vi "Init Plot.vi"(8 "error in":errorcluster, 11 "XYGraph in":refnum<vi>) -> (0 "error out":errorcluster)   [LabVIEW 2013, in "Display Data.lvclass"]
uses:
  Display Data.lvclass
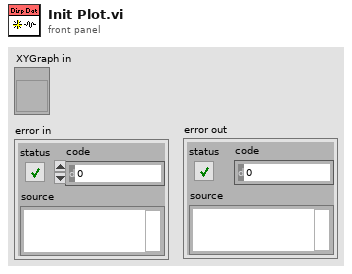
[diagram p1: front panel]
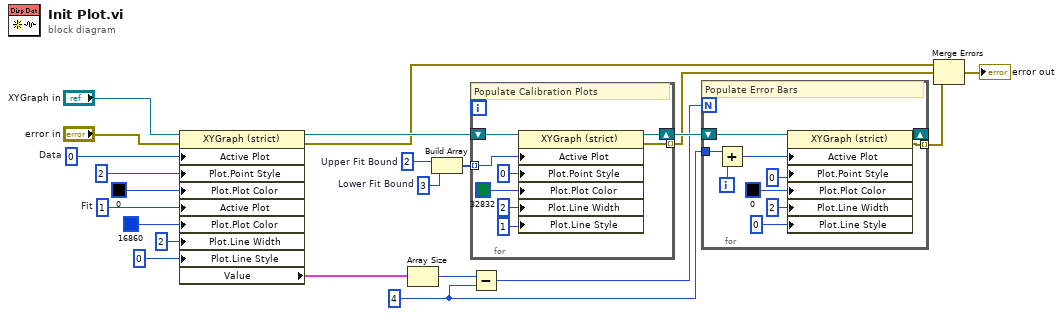
[diagram p0: block diagram]
diagram:
  w7 = 4 ("y")
  w19 = u32 3  # Lower Fit Bound
  w20 = u32 2  # Upper Fit Bound
  w13 = u32 1  # Fit
  w10 = u32 0  # Data
  n1 = property on="Property Node" class="XYGraph (strict)"(reference="XYGraph in", error in="error in", "Active Plot"=w10, "Plot.Point Style"=u8 2, "Plot.Plot Color"=u32 0, "Active Plot"=w13, "Plot.Plot Color"=u32 16860, "Plot.Line Width"=u8 2, "Plot.Line Style"=u8 0) -> (reference out=w18:refnum<vi>, error out=w3:errorcluster, "Value"=w9:cluster{dbl[], "Best Linear Fit":dbl[]}[])
  n2 = Array Size(array=w9) -> (size(s)=w8:i32)
  n3 = Build Array(w20, w19) -> (w21:u32[])
  n4 = for {
    shift-right: [w24] -> w22
    shift-left: w18 -> [w25]
    tunnel: w21 -> [w30] mode=indexing
    tunnel: [w23] -> w4 mode=indexing
    # "Populate Calibration Plots"
    n5 = property on="Property Node" class="XYGraph (strict)"(reference=w25, "Active Plot"=w30, "Plot.Point Style"=u8 0, "Plot.Plot Color"=u32 32832, "Plot.Line Width"=u8 2, "Plot.Line Style"=u8 1) -> (reference out=w24:refnum<vi>, error out=w23:errorcluster)  [unwired: 1 in]
  }
  n6 = Subtract(x=w8, y=w7) -> (x-y=w6:i32)
  n7 = for {
    N: w6 -> [_]
    shift-right: [w35] -> _
    shift-left: w22 -> [w36]
    tunnel: w7 -> [w33]
    tunnel: [w31] -> w5 mode=indexing
    i -> [w34]
    # "Populate Error Bars"
    n8 = Add(x=w33, y=w34) -> (x+y=w32:i32)
    n9 = property on="Property Node" class="XYGraph (strict)"(reference=w36, "Active Plot"=w32, "Plot.Point Style"=u8 0, "Plot.Plot Color"=u32 0, "Plot.Line Width"=u8 2, "Plot.Line Style"=u8 0) -> (reference out=w35:refnum<vi>, error out=w31:errorcluster)  [unwired: 1 in]
  }
  n10 = Merge Errors(w3, w4, w5) -> (→"error out":errorcluster)
